vi "Login.vi"() -> ()   [LabVIEW 2010]
doc: "A sample VI used to demonstrate different data types in LabVIEW, using a Login interface."
panel:
  out "Boolean":bool
  out "String":string
  in  "Password":string
  in  "Username":string
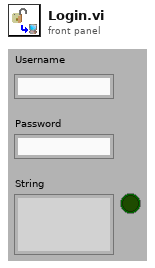
[diagram p1: front panel]
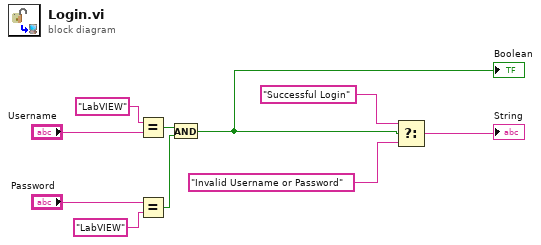
[diagram p0: block diagram]
diagram:
  n1 = Equal?(x="LabVIEW", y="Username") -> (x = y?=w6:bool)
  n2 = Equal?(x="Password", y="LabVIEW") -> (x = y?=w5:bool)
  n3 = And(x=w6, y=w5) -> (x .and. y?=w1:bool)
  "Boolean" <- w1
  n4 = Select(t="Successful Login" ("String"), s=w1, f="Invalid Username or Password") -> (s? t:f=→"String":string)
